vi "Stream Splitter.vi"(9 "Array lengh":i32, 10 "Ending edges":i32[](array[numeric]), 11 "Starting edges":i32[](array[numeric])) -> (3 "Segments":T1[](array[typedef]))   [LabVIEW 2016]
uses:
  Stream Segment.ctl
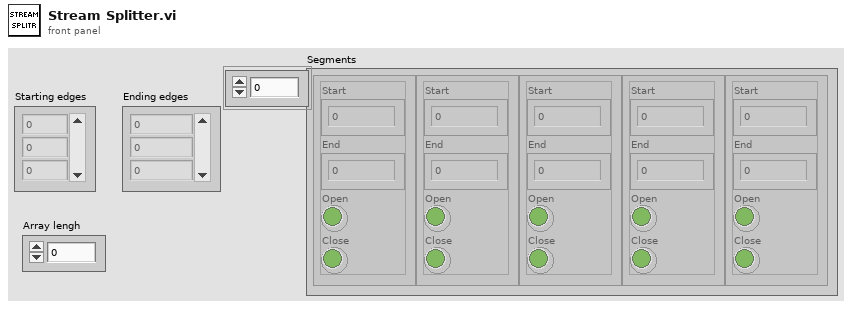
[diagram p1: front panel]
types:
  T1 = typedef "Stream Segment.ctl" = cluster{"Start":i32, "End":i32, "Open":bool, "Close":bool}
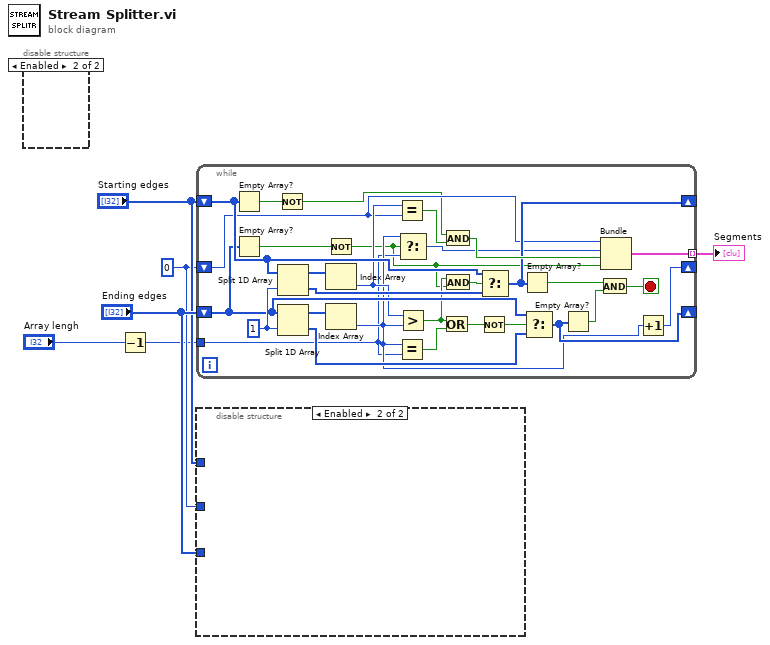
[diagram p0: block diagram]
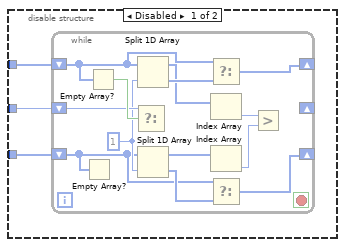
[diagram p2: hidden frame]
diagram:
  w4 = 0
  n1 = disable-structure shown="Enabled" {
    frame Disabled {
    }
    frame Enabled {
    }
  }
  n2 = Decrement(x="Array lengh") -> (x-1=w1:i32)
  n3 = while {
    shift-right: [w26] -> _
    shift-left: "Starting edges" -> [w36]
    shift-right: [w25] -> _
    shift-left: "Ending edges" -> [w30]
    shift-right: [w17] -> _
    shift-left: w4 -> [w18]
    tunnel: w1 -> [w9]
    tunnel: [w19] -> w2 mode=indexing
    stop <- w20 stop-if-true
    w31 = 1 ("index")
    n4 = Empty Array?(array=w36) -> (empty?=w29:bool)
    n5 = Empty Array?(array=w30) -> (empty?=w16:bool)
    n6 = Not(x=w29) -> (.not. x?=w11:bool)
    n7 = Split 1D Array(array=w36, index=w31) -> (first subarray=w34:i32[], second subarray=w35:i32[])
    n8 = Split 1D Array(array=w30, index=w31) -> (first subarray=w33:i32[], second subarray=w32:i32[])
    n9 = Not(x=w16) -> (.not. x?=w7:bool)
    n10 = Index Array(array=w34) -> (element=w28:i32)  [unwired: 1 in]
    n11 = Index Array(array=w33) -> (element=w10:i32)  [unwired: 1 in]
    n12 = Equal?(x=w28, y=w18) -> (x = y?=w14:bool)
    n13 = Equal?(x=w10, y=w9) -> (x = y?=w24:bool)
    n14 = Select(t=w10, s=w7, f=w9) -> (s? t:f=w8:i32)
    n15 = Greater?(x=w28, y=w10) -> (0:w13:bool)
    n16 = Or(x=w13, y=w24) -> (x .or. y?=w23:bool)
    n17 = And(x=w11, y=w14) -> (x .and. y?=w27:bool)
    n18 = And(x=w13, y=w7) -> (x .and. y?=w12:bool)
    n19 = Not(x=w23) -> (.not. x?=w15:bool)
    n20 = Select(t=w36, s=w12, f=w35) -> (s? t:f=w26:i32[])
    n21 = Empty Array?(array=w26) -> (empty?=w22:bool)
    n22 = Select(t=w30, s=w15, f=w32) -> (s? t:f=w25:i32[])
    n23 = Empty Array?(array=w25) -> (empty?=w21:bool)
    n24 = And(x=w22, y=w21) -> (x .and. y?=w20:bool)
    n25 = Bundle(w18, "Numeric"=w8, w27, w7) -> (w19:cluster{i32, "Numeric":i32, bool, bool})  [unwired: 1 in]
    n26 = Increment(x=w10) -> (x+1=w17:i32)
  }
  "Segments" <- w2
  n27 = disable-structure shown="Enabled" {
    disable-tunnel: "Ending edges" -> [w39 _]
    disable-tunnel: "Starting edges" -> [w38 _]
    disable-tunnel: w4 -> [w37 _]
    frame Disabled {
      n28 = while {
        shift-right: [w48] -> _
        shift-left: w38 -> [w50]
        shift-right: [w43] -> _
        shift-left: w39 -> [w40]
        shift-right: _ -> [_]
        shift-left: w37 -> [w51]
        stop <- _ stop-if-true
        w44 = 1 ("index")
        n29 = Empty Array?(array=w40) -> ()  [unwired: 1 out]
        n30 = Empty Array?(array=w50) -> (empty?=w52:bool)
        n31 = Select(t=w51, s=w52) -> ()  [unwired: 1 in, 1 out]
        n32 = Split 1D Array(array=w50, index=w44) -> (first subarray=w47:i32[], second subarray=w49:i32[])
        n33 = Split 1D Array(array=w40, index=w44) -> (first subarray=w46:i32[], second subarray=w45:i32[])
        n34 = Select(t=w50, f=w49) -> (s? t:f=w48:i32[])  [unwired: 1 in]
        n35 = Index Array(array=w47) -> (element=w42:i32)  [unwired: 1 in]
        n36 = Index Array(array=w46) -> (element=w41:i32)  [unwired: 1 in]
        n37 = Select(t=w40, f=w45) -> (s? t:f=w43:i32[])  [unwired: 1 in]
        n38 = Greater?(x=w42, y=w41) -> ()  [unwired: 1 out]
      }
    }
    frame Enabled {
    }
  }
